vi "Open Tank Drive.vi"() -> (0 "error out":errorcluster, 1 "navX Device":T1={"Interface"={"Protocol"=enum."SERIAL", "Update Rate (4Hz-60Hz)"=4, "navX Open TypeDef"=variant}, "Notify Packet"=refnum, "Loop VI Refnum"=refnum, "Ready to Close Occurrence Refnum"=refnum} {"Interface"."Update Rate (4Hz-60Hz)" min=4 max=60 step=1}, 2 "RobotDriveDevRef":T3={"DevStatus"={"status"=FALSE, "code"=0, "source"=""}, "Motors[]"=[], "Square Inputs"=FALSE, "Max Output"=1.0})   [LabVIEW 2015]
uses:
  <vilib>/Rock Robotics/WPI/RobotDrive/WPI_RobotDriveDevRef.ctl
  <vilib>/Rock Robotics/WPI/MotorControl/WPI_MotorControlDeviceRef.ctl
  <vilib>/Rock Robotics/WPI/MotorControl/WPI_MotorControlType.ctl
  <vilib>/Rock Robotics/SystemInterfaces/DIO/FPGA_DIOPWMChannel.ctl
  <vilib>/Rock Robotics/WPI/PWM/WPI_PWMDeadband.ctl
  <vilib>/Rock Robotics/WPI/CAN/Jaguar/SubVIs/WPI_CANJaguar_ControlMode.ctl
  <vilib>/Rock Robotics/WPI/CAN/TalonSRX/WPI_CANTalonSRX_APIControlMode.ctl
  Support Code/Team900-VIs/navX Library v2/TypeDefs/Z900_navX_DeviceTypeDef.ctl
  Support Code/Team900-VIs/navX Library v2/TypeDefs/Z900_navX_ProtocolTypeDef.ctl
  Support Code/Team900-VIs/navX Library v2/TypeDefs/Z900_navX_NotifyPacketTypeDef.ctl
  Support Code/Team900-VIs/navX Library v2/TypeDefs/Z900_navX_ActionTypeDef.ctl
  <vilib>/Rock Robotics/WPI/SafetyOutput/WPI_SafetyOutputConfigMenu.ctl
  <vilib>/Rock Robotics/WPI/CAN/TalonSRX/WPI_CANTalonSRX_APIFeedbackSelect.ctl
  <vilib>/Rock Robotics/SystemInterfaces/spilib/spi_bus.ctl
  <vilib>/Rock Robotics/WPI/MotorControl/WPI_MotorControlOpenCANTalonSRX.vi
  <vilib>/Rock Robotics/WPI/RobotDrive/WPI_RobotDriveOpen2MotorWithExistingMotors.vi
  Support Code/Team900-VIs/navX Library v2/IO/Open/Z900_navX_Open_SPI.vi
  Support Code/Team900-VIs/navX Library v2/navX Library v2.lvlib
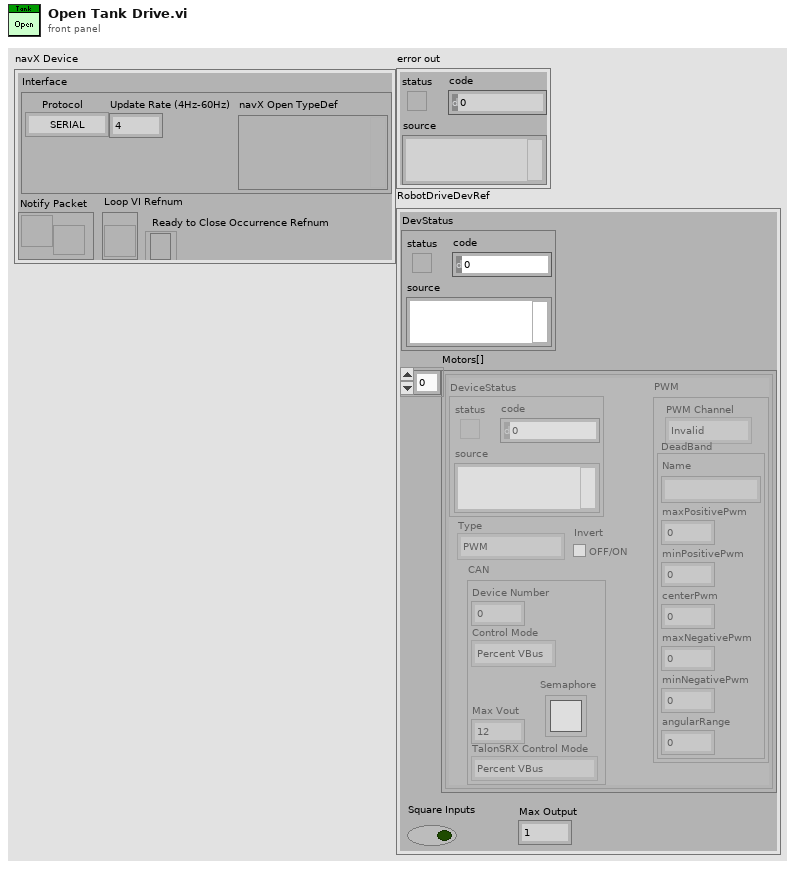
[diagram p1: front panel]
types:
  T1 = typedef "navX Library v2.lvlib/Z900_navX_DeviceTypeDef.ctl" = cluster{"Interface":cluster{"Protocol":T2, "Update Rate (4Hz-60Hz)":u8, "navX Open TypeDef":variant}, "Notify Packet":refnum<notifier>, "Loop VI Refnum":refnum<vi>, "Ready to Close Occurrence Refnum":refnum<k4>}
  T2 = typedef "navX Library v2.lvlib/Z900_navX_ProtocolTypeDef.ctl" = enum16{"SERIAL", "I2C", "SPI"}
  T3 = typedef "WPI_RobotDriveDevRef.ctl" = cluster{"DevStatus":errorcluster, "Motors[]":T4[], "Square Inputs":bool, "Max Output":dbl}
  T4 = typedef "WPI_MotorControlDeviceRef.ctl" = cluster{"DeviceStatus":errorcluster, "Type":T5, "PWM":cluster{"PWM Channel":T6, "DeadBand":T7}, "CAN":cluster{"Device Number":u8, "Control Mode":T8, "Semaphore":T9, "Max Vout":dbl, "TalonSRX Control Mode":T10}, "Invert":bool}
  T5 = typedef "WPI_MotorControlType.ctl" = enum16{"PWM", "CAN", "CANTalonSRX"}
  T6 = typedef "FPGA_DIOPWMChannel.ctl" = enum8{"PWM 0", "PWM 1", "PWM 2", "PWM 3", "PWM 4", "PWM 5", "PWM 6", "PWM 7", "PWM 8", "PWM 9", "PWM MXP 0", "PWM MXP 1", "PWM MXP 2", "PWM MXP 3", "PWM MXP 4", "PWM MXP 5", "PWM MXP 6", "PWM MXP 7", "PWM MXP 8", "PWM MXP 9", "Invalid"}
  T7 = typedef "WPI_PWMDeadband.ctl" = cluster{"Name":string, "maxPositivePwm":i32, "minPositivePwm":i32, "centerPwm":i32, "maxNegativePwm":i32, "minNegativePwm":i32, "angularRange":u16}
  T8 = typedef "WPI_CANJaguar_ControlMode.ctl" = enum8{"Percent VBus", "Current", "Speed", "Position", "Voltage"}
  T9 = typedef "Semaphore RefNum" = refnum<k1>
  T10 = typedef "WPI_CANTalonSRX_APIControlMode.ctl" = enum8{"Percent VBus", "Speed", "Position", "Slave", "Unchanged / Invalid", "Voltage Compensation", "Current", "Motion Profile"}
  T11 = typedef "WPI_CANTalonSRX_APIFeedbackSelect.ctl" = enum16{"Digital Quadrature Encoder", "Analog Potentiometer", "Analog Encoder", "Count on Quad-A (Rising-Edge)", "Count on Quad-A (Falling-Edge)", "CTR Magnetic Enc (Absolute)", "CTR Magnetic Enc (Relative)", "Pulse Width"}
  T12 = typedef "WPI_SafetyOutputConfigMenu.ctl" = enum16{"Enable", "Disable"}
  T13 = typedef "spi_bus.ctl" = enum16{"SPI On-Board, CS0", "SPI On-Board, CS1", "SPI On-Board, CS2", "SPI On-Board, CS3", "SPI MXP", "Invalid"}
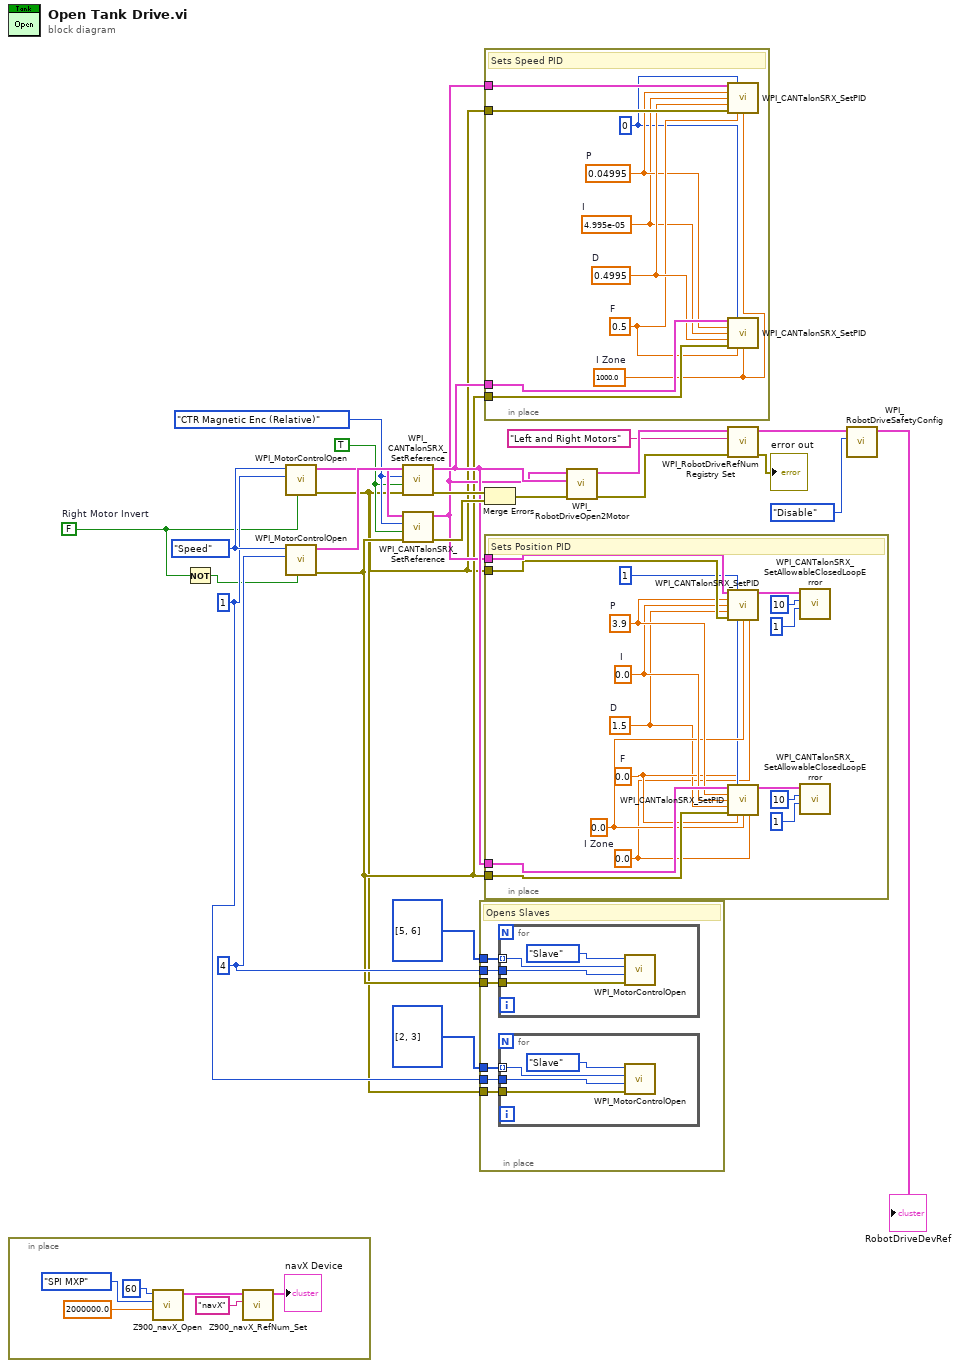
[diagram p0: block diagram]
diagram:
  w7 = TRUE ("Reverse Feedback Sensor")
  w9 = WPI_CANTalonSRX_APIFeedbackSelect."CTR Magnetic Enc (Relative)" ("Feedback Reference")
  w16 = FALSE  # Right Motor Invert
  w19 = u8 4 ("Device Number")
  w20 = u8 1 ("Device Number")
  w21 = WPI_CANTalonSRX_APIControlMode."Speed" ("Control Mode")
  n1 = in-place {
    n2 = call-poly "Z900_navX_Open.vi"("Clock Rate (Hz)"=2000000.0, "SPI Bus"=spi_bus."SPI MXP", "Update Rate (4Hz-60Hz)"=u8 60) -> ("navX Device"=w30:T1)  [unwired: 7 in, 1 out]
    n3 = call "Z900_navX_RefNum_Set.vi"("refnum name"="navX", "navX Device"=w30) -> ("navX Device"=→"navX Device":T1)  [unwired: 8 in, 1 out]
  }
  n4 = Not(x=w16) -> (.not. x?=w15:bool)
  n5 = call-poly <vilib>:"WPI_MotorControlOpen.vi"("Invert"=w16, "Device Number"=w20, "Control Mode"=w21) -> ("error out"=w2:errorcluster, "MotorControlDeviceRef"=w13:T4)  [unwired: 7 in]
  n6 = call-poly <vilib>:"WPI_MotorControlOpen.vi"("Invert"=w15, "Device Number"=w19, "Control Mode"=w21) -> ("error out"=w3:errorcluster, "MotorControlDeviceRef"=w14:T4)  [unwired: 7 in]
  n7 = call <vilib>:"WPI_CANTalonSRX_SetReference.vi"("error in (no error)"=w2, "Reverse Feedback Sensor"=w7, "Feedback Reference"=w9, "CAN Talon SRX Ref"=w14) -> ("error out"=w12:errorcluster, "CAN Talon SRX Ref"=w5:T4)  [unwired: 6 in]
  n8 = call <vilib>:"WPI_CANTalonSRX_SetReference.vi"("error in (no error)"=w3, "Reverse Feedback Sensor"=w7, "Feedback Reference"=w9, "CAN Talon SRX Ref"=w13) -> ("error out"=w11:errorcluster, "CAN Talon SRX Ref"=w4:T4)  [unwired: 6 in]
  n9 = in-place {
    in-place-border: w20 -> [w37]
    in-place-border: w19 -> [w36]
    in-place-border: u8[] [2, 3] -> [w35]
    in-place-border: u8[] [5, 6] -> [w34]
    in-place-border: w3 -> [w33]
    in-place-border: w2 -> [w32]
    # "Opens Slaves"
    n10 = for {
      tunnel: w36 -> [w41]
      tunnel: w34 -> [w39] mode=indexing
      tunnel: w33 -> [w38]
      n11 = call-poly <vilib>:"WPI_MotorControlOpen.vi"("error in (no error)"=w38, "Master Device Number"=w41, "Device Number"=w39, "Control Mode"=WPI_CANTalonSRX_APIControlMode."Slave") -> ()  [unwired: 6 in, 2 out]
    }
    n12 = for {
      tunnel: w37 -> [w45]
      tunnel: w35 -> [w43] mode=indexing
      tunnel: w32 -> [w42]
      n13 = call-poly <vilib>:"WPI_MotorControlOpen.vi"("error in (no error)"=w42, "Master Device Number"=w45, "Device Number"=w43, "Control Mode"=WPI_CANTalonSRX_APIControlMode."Slave") -> ()  [unwired: 6 in, 2 out]
    }
  }
  n14 = in-place {
    in-place-border: w5 -> [w55]
    in-place-border: w4 -> [w54]
    in-place-border: w3 -> [w53]
    in-place-border: w2 -> [w52]
    w46 = u8 0 ("Parameter Slot")
    w47 = 1000.0  # I Zone
    w50 = 0.5  # F
    w51 = 0.4995  # D
    w48 = 4.995e-05  # I
    w49 = 0.04995  # P
    # "Sets Speed PID"
    n15 = call <vilib>:"WPI_CANTalonSRX_SetPID.vi"("CAN Talon SRX Ref"=w54, "Parameter Slot"=w46, "P"=w49, "I"=w48, "D"=w51, "error in (no error)"=w52, "F"=w50, "I Zone"=w47) -> ()  [unwired: 6 in, 2 out]
    n16 = call <vilib>:"WPI_CANTalonSRX_SetPID.vi"("CAN Talon SRX Ref"=w55, "Parameter Slot"=w46, "P"=w49, "I"=w48, "D"=w51, "error in (no error)"=w53, "F"=w50, "I Zone"=w47) -> ()  [unwired: 6 in, 2 out]
  }
  n17 = Merge Errors(w12, w11) -> (w10:errorcluster)
  n18 = in-place {
    in-place-border: w5 -> [w72]
    in-place-border: w4 -> [w71]
    in-place-border: w3 -> [w70]
    in-place-border: w2 -> [w69]
    w56 = 0.0 ("Ramp Rate")
    w65 = u8 1 ("Parameter Slot")
    w66 = 0.0  # I Zone
    w64 = 0.0  # F
    w57 = 1.5  # D
    w67 = 0.0  # I
    w68 = 3.9  # P
    # "Sets Position PID"
    n19 = call <vilib>:"WPI_CANTalonSRX_SetPID.vi"("CAN Talon SRX Ref"=w71, "Parameter Slot"=w65, "P"=w68, "I"=w67, "D"=w57, "error in (no error)"=w69, "F"=w64, "I Zone"=w66, "Ramp Rate"=w56) -> ("CAN Talon SRX Ref"=w58:T4)  [unwired: 5 in, 1 out]
    n20 = call <vilib>:"WPI_CANTalonSRX_SetPID.vi"("CAN Talon SRX Ref"=w72, "Parameter Slot"=w65, "P"=w68, "I"=w67, "D"=w57, "error in (no error)"=w70, "F"=w64, "I Zone"=w66, "Ramp Rate"=w56) -> ("CAN Talon SRX Ref"=w61:T4)  [unwired: 5 in, 1 out]
    n21 = call <vilib>:"WPI_CANTalonSRX_SetAllowableClosedLoopError.vi"("Parameter Slot"=u8 1, "Allowable Closed-Loop Error"=u16 10, "CAN Talon SRX Ref"=w58) -> ()  [unwired: 7 in, 2 out]
    n22 = call <vilib>:"WPI_CANTalonSRX_SetAllowableClosedLoopError.vi"("Parameter Slot"=u8 1, "Allowable Closed-Loop Error"=u16 10, "CAN Talon SRX Ref"=w61) -> ()  [unwired: 7 in, 2 out]
  }
  n23 = call-poly <vilib>:"WPI_RobotDriveOpen2Motor.vi"("error in (no error)"=w10, "Right Motor Dev Ref"=w5, "Left Motor Dev Ref"=w4) -> ("error out"=w8:errorcluster, "RobotDriveDevRef"=w25:T3)  [unwired: 2 in, 5 out]
  n24 = call <vilib>:"WPI_RobotDriveRefNum Registry Set.vi"("error in (no error)"=w8, "refnum name"="Left and Right Motors", "RobotDriveDevRef"=w25) -> ("error out"=→"error out":errorcluster, "RobotDriveDevRef"=w23:T3)  [unwired: 1 in, 6 out]
  n25 = call <vilib>:"WPI_RobotDriveSafetyConfig.vi"("mode"=WPI_SafetyOutputConfigMenu."Disable", "RobotDriveDevRef"=w23) -> ("RobotDriveDevRef"=→"RobotDriveDevRef":T3)  [unwired: 8 in, 1 out]
